vi "Read Configuration File.vi"(8 "error in (no error)":errorcluster, 11 "Example Instrument in":refnum<class "LevyLab Instrument.lvclass">) -> (0 "error out":errorcluster, 3 "Example Instrument out":refnum<class "LevyLab Instrument.lvclass">)   [LabVIEW 2016, in "LevyLab Instrument.lvclass"]
uses:
  LevyLab Instrument.lvclass
  C:/user/patrick/git/Instrument-Framework/lvsrc/SMOs/Instrument/Instrument.lvclass
  SMOs/Instrument/Instrument.lvclass/Instrument.ctl
  LevyLab Instrument.lvclass/LevyLab Instrument.ctl
  SMOs/Configuration/Configuration.lvclass
  SMOs/Instrument/Instrument.lvclass
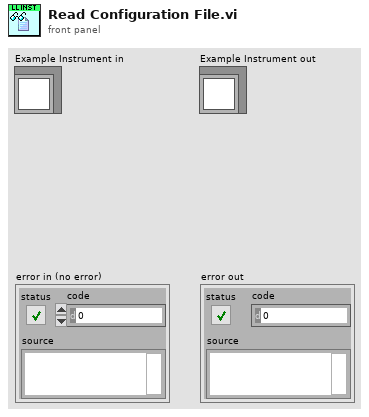
[diagram p1: front panel]
types:
  T1 = typedef "LevyLab Instrument.lvclass/LevyLab Instrument.Configuration--Cluster.ctl" = cluster{"Example Setting 1":dbl, "Example Setting 2":dbl, "Example Setting 3":string}
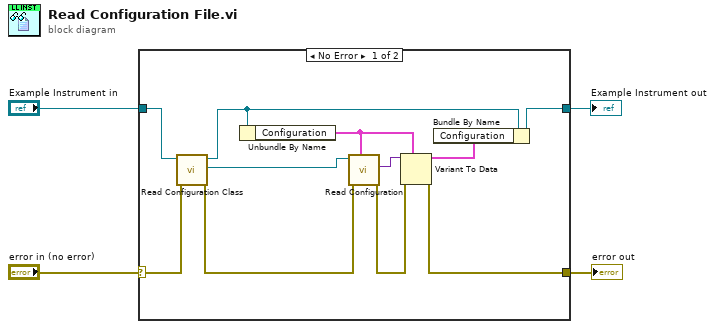
[diagram p0: block diagram]
diagram:
  n1 = case shown="No Error" "error in (no error)" {
    selector: "error in (no error)" -> [w8 w17]
    tunnel: "Example Instrument in" -> [w11 w16]
    tunnel: [w6 w16] -> w3
    tunnel: [w9 w17] -> w2
    frame No Error {
      n2 = call "Read Configuration Class.vi"("error in (no error)"=w8, "Instrument in"=w11) -> ("error out"=w12:errorcluster, "Configuration.lvclass"=w13:refnum<class "Configuration.lvclass">, "Instrument out"=w5:refnum<class "LevyLab Instrument.lvclass">)  [unwired: 7 in]
      n3 = Unbundle By Name(w5) -> ("Configuration"=w7:T1)
      n4 = call "Read Configuration.vi"("INI Fomatted Cluster Type"=w7, "error in (no error)"=w12, "Configuration in"=w13) -> ("error out"=w14:errorcluster, "Configuration"=w15:variant)  [unwired: 6 in, 1 out]
      n5 = Variant To Data(error in=w14, type=w7, Variant=w15) -> (data=w10:T1, error out=w9:errorcluster)
      n6 = Bundle By Name(cluster=w5, "Configuration"=w10) -> (w6:refnum<class "LevyLab Instrument.lvclass">)
    }
    frame Error {
    }
  }
  "Example Instrument out" <- w3
  "error out" <- w2
